vi "Global-Find System.vi"(11 "VISA session":refnum<visa-resource-name>) -> (0 "found":bool, 1 "active error checking":bool, 2 "SMU6 present":bool, 3 "VISA resource name out":refnum<visa-resource-name>, 4 "PGU2 present":bool, 5 "PGU1 present":bool, 6 "GNDU present":bool, 7 "SMU5 present":bool)   [LabVIEW 2016, in "Agilent 415X Series.lvlib"]
doc: "This VI uses an instrment's \"instrument handler\" as a key to search for the instrument's system configuration (extra models) in global data structures."
uses:
  Agilent 415X Series.lvlib
  Private/Global.vi
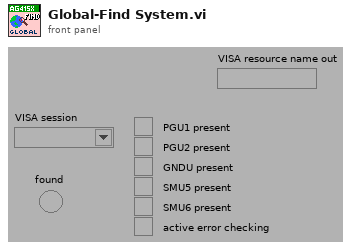
[diagram p1: front panel]
types:
  T1 = cluster{"valid instrument":bool, "GNDU present":bool, "SMU5 present":bool, "SMU6 present":bool, "PGU1 present":bool, "PGU2 present":bool, "active error checking":bool, "instr. handler":refnum<visa-resource-name>}[]
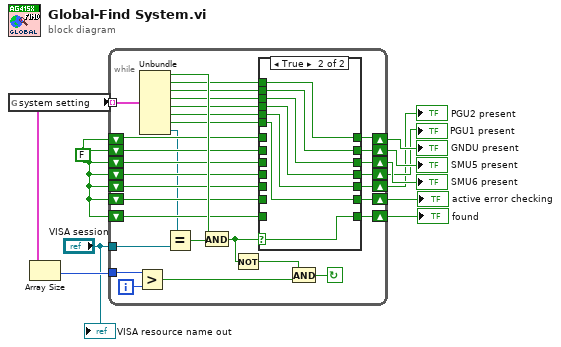
[diagram p0: block diagram]
diagram:
  w2 = FALSE
  n1 = global read "Global.vi" "system setting"() -> (w8:T1)
  n2 = Array Size(array=w8) -> (size(s)=w11:i32)
  n3 = while {
    shift-left: w2 -> [w15]
    shift-right: [w14] -> w1
    shift-left: w2 -> [w17]
    shift-right: [w16] -> w7
    shift-left: w2 -> [w24]
    shift-right: [w19] -> w10
    shift-left: w2 -> [w25]
    shift-right: [w20] -> w3
    shift-left: w2 -> [w26]
    shift-right: [w21] -> w4
    shift-left: w2 -> [w27]
    shift-right: [w22] -> w5
    shift-left: w2 -> [w28]
    shift-right: [w23] -> w6
    tunnel: w11 -> [w38]
    tunnel: "VISA session" -> [w41]
    tunnel: w8 -> [w42] mode=indexing
    i -> [w37]
    stop <- w35 continue-if-true
    n4 = Greater?(x=w38, y=w37) -> (0:w36:bool)
    n5 = Unbundle(w42) -> ("valid instrument"=w40:bool, "GNDU present"=w34:bool, "SMU5 present"=w33:bool, "SMU6 present"=w32:bool, "PGU1 present"=w31:bool, "PGU2 present"=w18:bool, "active error checking"=w12:bool, "instr. handler"=w13:refnum<visa-resource-name>)
    n6 = Equal?(x=w13, y=w41) -> (x = y?=w39:bool)
    n7 = And(x=w40, y=w39) -> (x .and. y?=w29:bool)
    n8 = Not(x=w29) -> (.not. x?=w30:bool)
    n9 = case shown="True" w29 {
      selector: w29 -> [_ w56]
      tunnel: w34 -> [_ w55]
      tunnel: w33 -> [_ w52]
      tunnel: w32 -> [_ w53]
      tunnel: w31 -> [_ w54]
      tunnel: w28 -> [w49 _]
      tunnel: w27 -> [w48 _]
      tunnel: w26 -> [w47 _]
      tunnel: w25 -> [w46 _]
      tunnel: w24 -> [w45 _]
      tunnel: [w49 w55] -> w23
      tunnel: [w48 w52] -> w22
      tunnel: [w47 w53] -> w21
      tunnel: [w46 w54] -> w20
      tunnel: [w45 w56] -> w19
      tunnel: w18 -> [_ w51]
      tunnel: w17 -> [w44 _]
      tunnel: [w44 w50] -> w16
      tunnel: w15 -> [w43 _]
      tunnel: [w43 w51] -> w14
      tunnel: w12 -> [_ w50]
      frame False {
      }
      frame True {
      }
    }
    n10 = And(x=w30, y=w36) -> (x .and. y?=w35:bool)
  }
  "found" <- w10
  "PGU1 present" <- w3
  "GNDU present" <- w6
  "SMU6 present" <- w4
  "SMU5 present" <- w5
  "active error checking" <- w7
  "PGU2 present" <- w1
  "VISA resource name out" <- "VISA session"
